vi "Save Buffer.vi"(6 "File Name(\"\")":string, 8 "error in (no error)":errorcluster, 9 "Information (4: All)":i32(ring)=4 items=["Format", "Relative", "Raw", "Stamp", "All", "Standard", "Brief", "Extra", "Status", "Chancol", "Easygraph"], 10 "Buffer Name (\"\")":string, 11 "VISA resource name":refnum<visa-resource-name>) -> (0 "error out":errorcluster, 3 "VISA resource name out":refnum<visa-resource-name>)   [LabVIEW 2015, in "Keithley DMM6500 DAQ6500 Series.lvlib"]
doc: "Save a buffer with corresponding information to disk."
uses:
  <instrlib>/Keithley DMM6500 DAQ6500 Series/Keithley DMM6500 DAQ6500 Series.lvlib
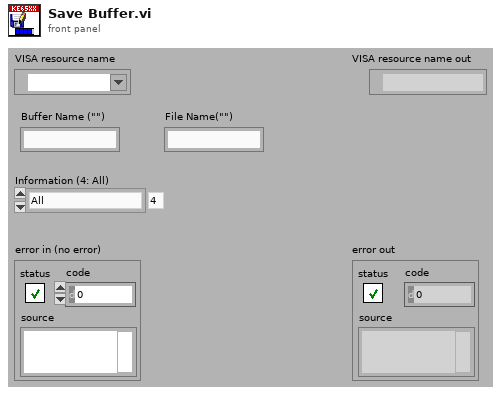
[diagram p1: front panel]
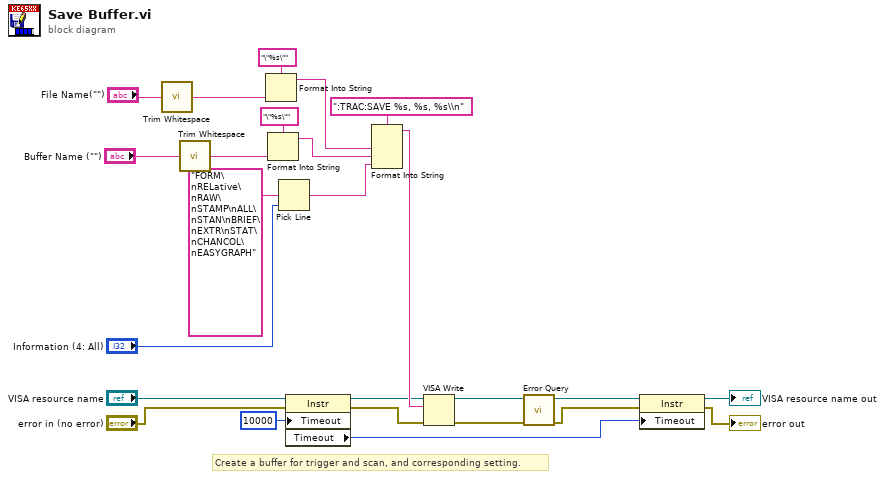
[diagram p0: block diagram]
diagram:
  # "Create a buffer for trigger and scan, and corresponding setting."
  n1 = call <vilib>:"Trim Whitespace.vi"("string"="File Name(\"\")") -> ("trimmed string"=w17:string)  [unwired: 1 in]
  n2 = call <vilib>:"Trim Whitespace.vi"("string"="Buffer Name (\"\")") -> ("trimmed string"=w15:string)  [unwired: 1 in]
  n3 = Format Into String(format string="\"%s\"", w17) -> (resulting string=w18:string)  [unwired: 2 in, 1 out]
  n4 = Format Into String(format string="\"%s\"", w15) -> (resulting string=w14:string)  [unwired: 2 in, 1 out]
  n5 = Pick Line(multi-line string="FORM\nRELative\nRAW\nSTAMP\nALL\nSTAN\nBRIEF\nEXTR\nSTAT\nCHANCOL\nEASYGRAPH", line index="Information (4: All)") -> (output string=w21:string)  [unwired: 1 in]
  n6 = property class="Instr"(reference="VISA resource name", error in="error in (no error)", "Timeout"=u32 10000 ("General Settings:Timeout Value")) -> (reference out=w8:refnum<visa-resource-name>, error out=w7:errorcluster, "Timeout"=w1:u32)
  n7 = Format Into String(format string=":TRAC:SAVE %s, %s, %s\\n", w18, w14, w21) -> (resulting string=w13:string)  [unwired: 2 in, 1 out]
  n8 = VISA Write(VISA resource name=w8, write buffer=w13, error in (no error)=w7) -> (VISA resource name out=w24:refnum<visa-resource-name>, error out=w23:errorcluster)  [unwired: 1 out]
  n9 = call <instrlib>:"Error Query.vi"("error in (no error)"=w23, "VISA resource name"=w24) -> ("error out"=w3:errorcluster, "VISA resource name out"=w5:refnum<visa-resource-name>)  [unwired: 6 in, 2 out]
  n10 = property class="Instr"(reference=w5, error in=w3, "Timeout"=w1) -> (reference out=→"VISA resource name out":refnum<visa-resource-name>, error out=→"error out":errorcluster)
